vi "U3 Clock Check.vi"() -> ()   [LabVIEW 2021]
panel:
  out "Sys Time, U3 Time, VS, LM34, PPM error":dbl[][](array[numeric]) format="%.2f"
  in  "error in":errorcluster
  in  "Address":string="1"
  in  "FirstFound":bool=TRUE
  in  "stop":bool
  out "error out":errorcluster
  out "Error Message":string
  # "This VI acquires the U3 system timer and the PC system timer, every 60 seconds, and calculates the \nU3 clock error in PPM assuming the PC clock is right.  The U3 clock is rated at just 1.5%,\nwhich is 15000 PPM.\n\nThis approach could likely be used to adjust the U3 clock readings to the accuracy of the\nPC clock, over a short term anyway.\n\nThis VI also acquires VS (jumpered to AIN0 on a U3-HV) and the voltage from an EI-1034\nor LM34 (on FIO5).  Device voltage and temperature are the 2 likely factors that would\naffect the system clock."
  # "This VI passes a timer\nbase clock constant that\nis valid for hardware V1.21.\nFor hardware V1.20 change\nLJ_tc48MHZ_DIV to LJ_tc24MHZ_DIV."
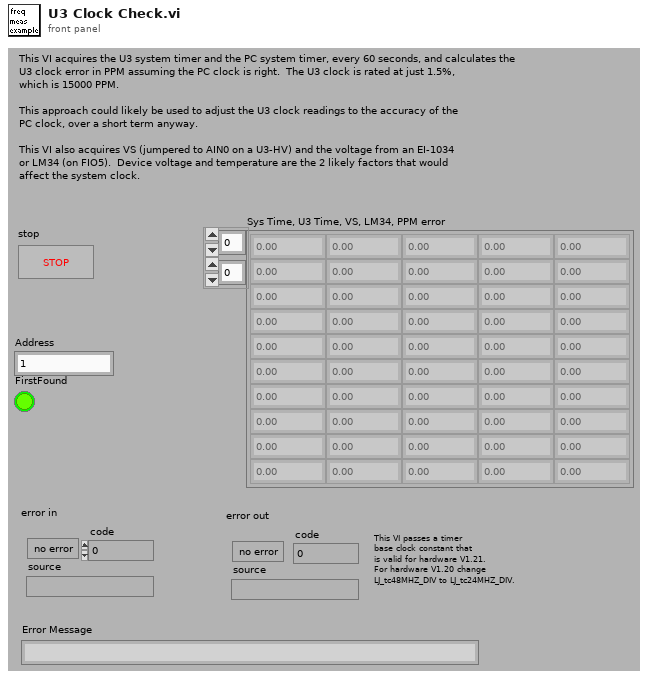
[diagram p1: front panel]
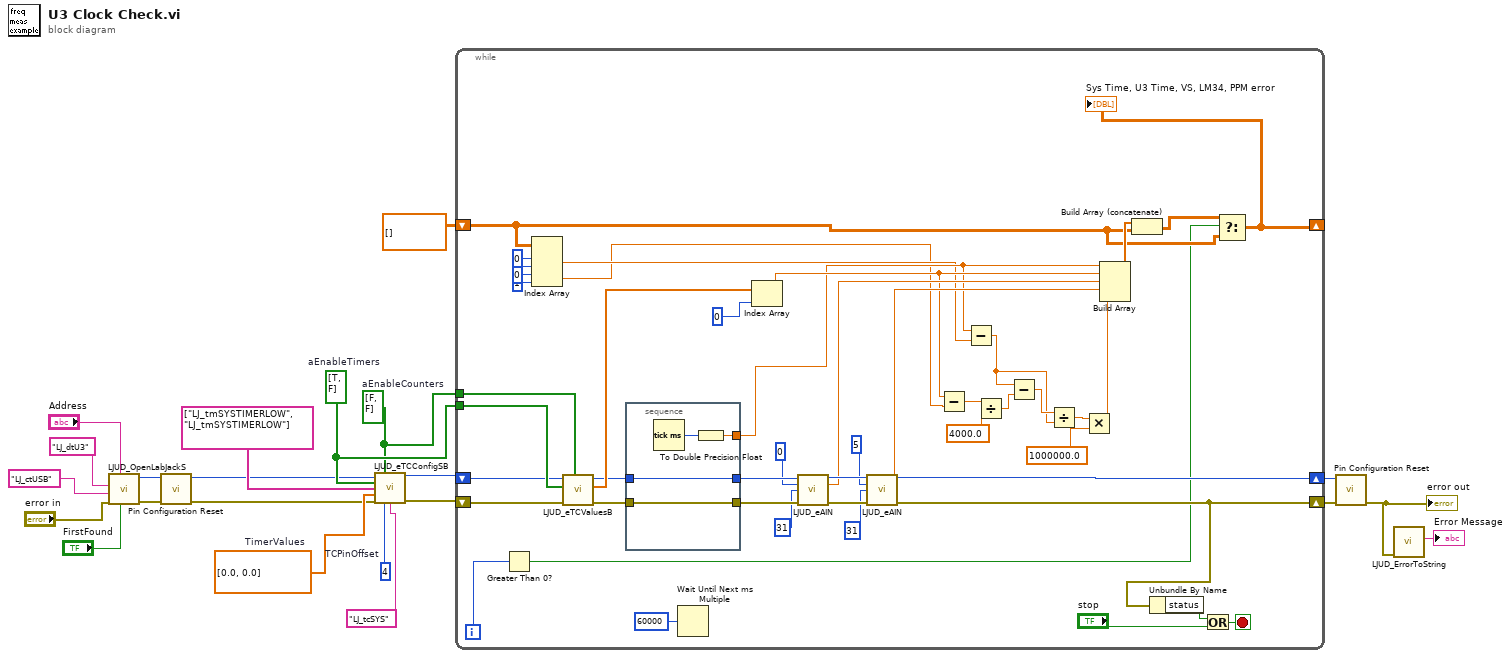
[diagram p0: block diagram]
diagram:
  w6 = 4  # TCPinOffset
  w11 = bool[] [FALSE, FALSE]  # aEnableCounters
  w12 = bool[] [TRUE, FALSE]  # aEnableTimers
  w15 = dbl[] [0.0, 0.0]  # TimerValues
  n1 = call "LJUD_OpenLabJackS.vi"("FirstFound"="FirstFound", "Address"="Address", "error in"="error in", "ConnectionType"="LJ_ctUSB", "DeviceType"="LJ_dtU3") -> ("error out"=w4:errorcluster, "Handle"=w5:i32)  [unwired: 4 in, 1 out]
  n2 = call "Pin Configuration Reset.vi"("error in"=w4, "Handle In"=w5) -> ("error out"=w2:errorcluster, "Handle Out"=w3:i32)  [unwired: 8 in]
  n3 = call "LJUD_eTCConfigSB.vi"("Handle In"=w3, "aEnableCounters"=w11, "aEnableTimers"=w12, "aTimerModes"=string[] ["LJ_tmSYSTIMERLOW", "LJ_tmSYSTIMERLOW"] ("TimerModes"), "aTimerValues"=w15, "error in"=w2, "TCPinOffset"=w6, "TimerClockBase"="LJ_tcSYS" ("Timer Clock Base")) -> ("Handle Out"=w17:i32, "error out"=w16:errorcluster)  [unwired: 6 in]
  n4 = while {
    shift-left: dbl[][] [] -> [w26]
    shift-right: [w25] -> _
    tunnel: w11 -> [w64]
    tunnel: w12 -> [w65]
    shift-left: w16 -> [w62]
    shift-right: [w57] -> w9
    shift-left: w17 -> [w63]
    shift-right: [w51] -> w10
    i -> [w24]
    stop <- w68 stop-if-true
    n5 = Greater Than 0?(x=w24) -> (x > 0?=w23:bool)
    n6 = Index Array(array=w26, index (row) #1=0 ("Index (row)"), index (col) #1=0 ("Disabled Index (col)"), index (row) #2=0 ("Index (row)"), index (col) #2=1 ("Disabled Index (col)")) -> (element #1=w33:dbl, element #2=w32:dbl)
    n7 = call "LJUD_eTCValuesB.vi"("aReadCounters"=w64, "error in"=w62, "aReadTimers"=w65, "Handle In"=w63) -> ("error out"=w60:errorcluster, "aTimerValues Read"=w55:dbl[], "Handle Out"=w54:i32)  [unwired: 4 in, 1 out]
    n8 = stacked-sequence {
      tunnel: w60 -> [w72]
      tunnel: [w72] -> w59
      tunnel: w54 -> [w71]
      tunnel: [w71] -> w53
      tunnel: [w70] -> w34
      frame #0 {
        n9 = Tick Count (ms)() -> (millisecond timer value=w69:u32)
        n10 = To Double Precision Float(number=w69) -> (double precision float=w70:dbl)
      }
    }
    n11 = Wait Until Next ms Multiple(millisecond multiple=u32 60000 ("milliseconds to wait")) -> ()  [unwired: 1 out]
    n12 = Index Array(array=w55, index=0 ("Index")) -> (element=w35:dbl)
    n13 = call "LJUD_eAIN.vi"("Handle In"=w53, "ChannelP"=0, "ChannelN"=31, "error in"=w59) -> ("Handle Out"=w52:i32, "Voltage"=w43:dbl, "error out"=w58:errorcluster)  [unwired: 9 in]
    n14 = call "LJUD_eAIN.vi"("Handle In"=w52, "ChannelP"=5, "ChannelN"=31, "error in"=w58) -> ("Handle Out"=w51:i32, "Voltage"=w42:dbl, "error out"=w57:errorcluster)  [unwired: 9 in]
    n15 = Subtract(x=w35, y=w32) -> (x-y=w31:dbl)
    n16 = Subtract(x=w34, y=w33) -> (x-y=w30:dbl)
    n17 = Divide(x=w31, y=4000.0) -> (x/y=w47:dbl)
    n18 = Subtract(x=w30, y=w47) -> (x-y=w46:dbl)
    n19 = Divide(x=w46, y=w30) -> (x/y=w45:dbl)
    n20 = Multiply(x=w45, y=1000000.0) -> (x*y=w41:dbl)
    n21 = Build Array(w34, w35, w43, w42, w41) -> (w40:dbl[])
    n22 = Build Array (concatenate)(w40, w26) -> (w27:dbl[][])
    n23 = Unbundle By Name(w57) -> ("status"=w67:bool)
    n24 = Or(x=w67, y="stop") -> (x .or. y?=w68:bool)
    n25 = Select(t=w27, s=w23, f=w26) -> (s? t:f=w25:dbl[][])
    "Sys Time, U3 Time, VS, LM34, PPM error" <- w25
  }
  n26 = call "Pin Configuration Reset.vi"("error in"=w9, "Handle In"=w10) -> ("error out"=w8:errorcluster)  [unwired: 8 in, 1 out]
  "error out" <- w8
  n27 = call "LJUD_ErrorToString.vi"("error in"=w8) -> ("String"=→"Error Message":string)  [unwired: 10 in]
